vi "Do.vi"(8 "error in (no error)":errorcluster, 10 "Actor in":refnum<class "Actor.lvclass">, 11 "Insert Bound View Msg":refnum<class "Insert Bound View Msg.lvclass">) -> (0 "error out":errorcluster, 2 "Actor out":refnum<class "Actor.lvclass">)   [LabVIEW 2018, in "MVA Framework.lvlib" / "BoundViewManager.lvlib" / "Insert Bound View Msg.lvclass"]
doc: "(<B>Filename</B>: Actor Framework.lvlib:Message.lvclass:Do.vi)\n\nDefines what a message does when it is received by an actor. Generally, a message instructs an actor to invoke one of its methods. By default, this method does nothing. A child class must override it to define behavior. Create a child class by using the Actor Framework Message Maker dialog box."
uses:
  Insert Bound View Msg.lvclass
  BoundViewManager/BoundViewManager.lvclass
  <vilib>/ActorFramework/Actor/Actor.lvclass
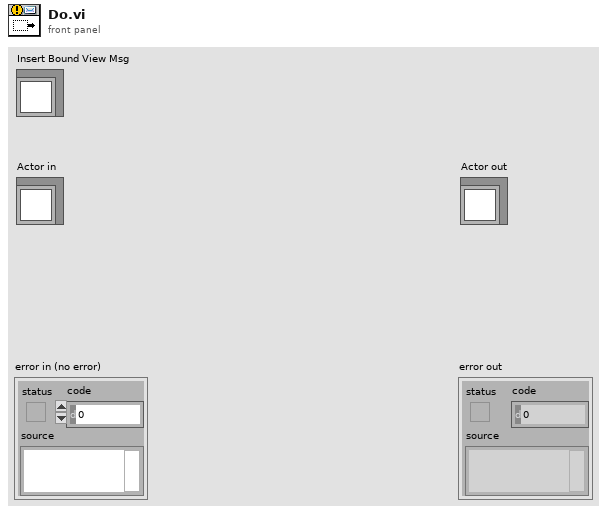
[diagram p1: front panel]
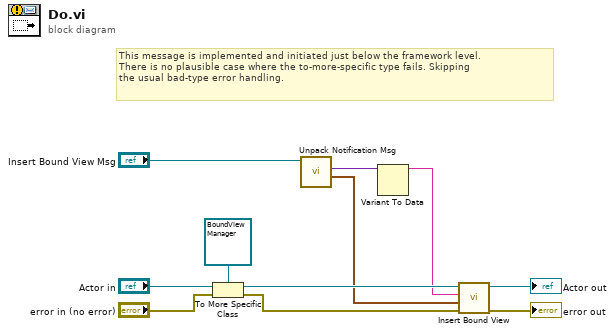
[diagram p0: block diagram]
diagram:
  # "This message is implemented and initiated just below the framework level.\nThere is no plausible case where the to-more-specific type fails. Skipping\nthe usual bad-type error handling."
  n1 = To More Specific Class(target class=refnum<class "BoundViewManager.lvclass"> refnum ("BoundViewManager.lvlib:BoundViewManager.lvclass"), reference="Actor in", error in="error in (no error)") -> (specific class reference=w8:refnum<class "BoundViewManager.lvclass">, error out=w6:errorcluster)
  n2 = call-dynamic "Unpack Notification Msg.vi"("Notification Msg"="Insert Bound View Msg") -> ("Publication Time"=w3:timestamp, "Value"=w2:variant)  [unwired: 8 in, 1 out]
  n3 = Variant To Data(Variant=w2) -> (data=w1:string)  [unwired: 2 in, 1 out]
  n4 = call-dynamic "Insert Bound View.vi"("error in (no error)"=w6, "Value Publication Time"=w3, "Selector Value"=w1, "BoundViewManager in"=w8) -> ("error out"=→"error out":errorcluster, "BoundViewManager out"=→"Actor out":refnum<class "BoundViewManager.lvclass">)  [unwired: 6 in]
